vi "Find Classes Out of Date.vi"(8 "error in (no error)":errorcluster, 11 "Test Finder In":refnum<class "Test Finder.lvclass">) -> (0 "error out":errorcluster, 2 "Outdated Test Class paths":path[](array[path]), 3 "Test Finder Out":refnum<class "Test Finder.lvclass">)   [LabVIEW 2020, in "Test Finder.lvclass"]
uses:
  Test Finder.lvclass
  Test Finder.lvclass/Test Finder.ctl
  Filter Test Cases.vi
  Find all Classes in LV XML.vi
  <vilib>/Utility/LVClass/Get LV Class Default Value.vi
  <vilib>/Utility/libraryn.llb/Recursive File List.vi
  LUnit Test Case.lvclass
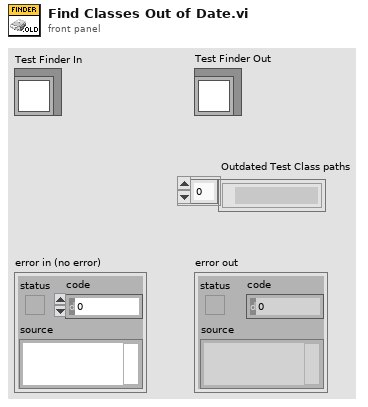
[diagram p1: front panel]
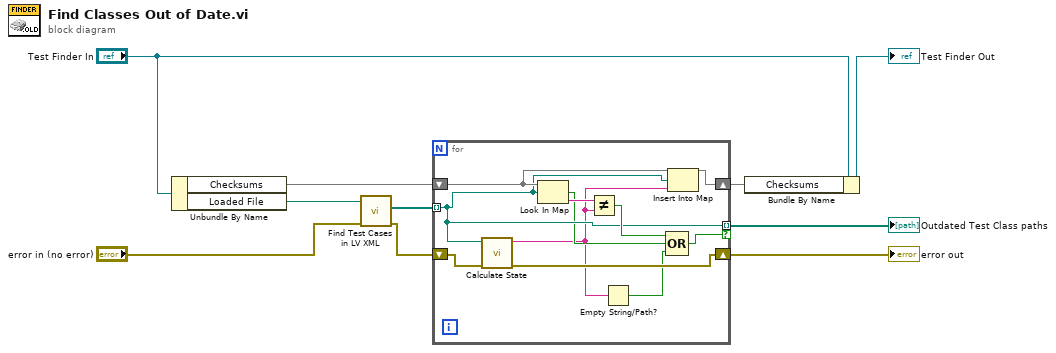
[diagram p0: block diagram]
diagram:
  n1 = Unbundle By Name("Test Finder In") -> ("Checksums"=w4:map{path, string}, "Loaded File"=w9:path)
  n2 = call "Find Test Cases in LV XML.vi"("error in (no error)"="error in (no error)", "Path"=w9) -> ("error out"=w6:errorcluster, "Test Class paths"=w7:path[])  [unwired: 8 in]
  n3 = for {
    tunnel: w7 -> [w15] mode=indexing
    shift-right: [w20] -> w5
    shift-left: w6 -> [w21]
    tunnel: [w15] -> w3 mode=indexing if=w14
    shift-right: [w16] -> w1
    shift-left: w4 -> [w17]
    n4 = call "Calculate State.vi"("error in (no error)"=w21, "Path"=w15) -> ("error out"=w20:errorcluster, "digest"=w12:string)  [unwired: 8 in]
    n5 = Look In Map(map=w17, key=w15) -> (key not found?=w13:bool, value=w19:string)  [unwired: 1 in]
    n6 = Not Equal?(x=w19, y=w12) -> (x != y?=w18:bool)
    n7 = Empty String/Path?(string/path=w12) -> (empty?=w11:bool)
    n8 = Compound Arithmetic op=OR(w18, w13, w11) -> (w14:bool)
    n9 = Insert Into Map(map in=w17, key=w15, value=w12) -> (map out=w16:map{path, string})  [unwired: 2 out]
  }
  "error out" <- w5
  "Outdated Test Class paths" <- w3
  n10 = Bundle By Name(cluster="Test Finder In", "Checksums"=w1) -> (→"Test Finder Out":refnum<class "Test Finder.lvclass">)
